vi "bmlv_tests_dict.vi"   [LabVIEW 2014]
uses:
  bmlv/Dictionary/Dictionary.lvclass
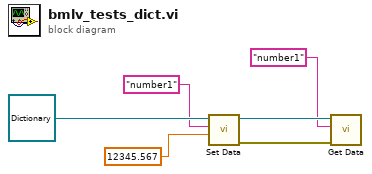
[diagram p0: block diagram]
diagram:
  n1 = call-dynamic "Set Data.vi"("Data"=12345.567, "Name"="number1", "Dictionary in"=refnum<class "Dictionary.lvclass"> refnum ("bmlv.lvlib:Dictionary.lvclass")) -> ("error out"=w1:errorcluster, "Dictionary out"=w3:refnum<class "Dictionary.lvclass">)  [unwired: 7 in]
  n2 = call-dynamic "Get Data.vi"("error in (no error)"=w1, "Name"="number1", "Dictionary in"=w3) -> ()  [unwired: 6 in, 3 out]
